vi "5-bit DIO.vi"(0 "DIO Refnum 1":refnum<k21>, 1 "DIO Refnum 2":refnum<k21>, 2 "DIO Refnum 3":refnum<k21>, 3 "DIO Refnum 4":refnum<k21>, 4 "DIO Refnum 5":refnum<k21>, 5 "DIO OUT[4:0]":u8, 7 "DIO DIR[4:0]":u8) -> (17 "DIO IN[4:0]":u8)   [LabVIEW 2019]
panel:
  # "This VI reads a Boolean value from or writes the value to the specified FPGA I/O item according to the direction of the data flow (DIR).\n- DIR: TRUE - Write data to OUT\n- DIR: FALSE - Read data from IN"
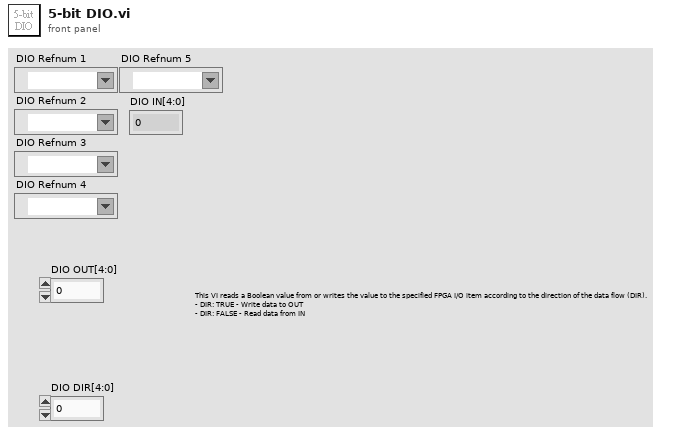
[diagram p1: front panel]
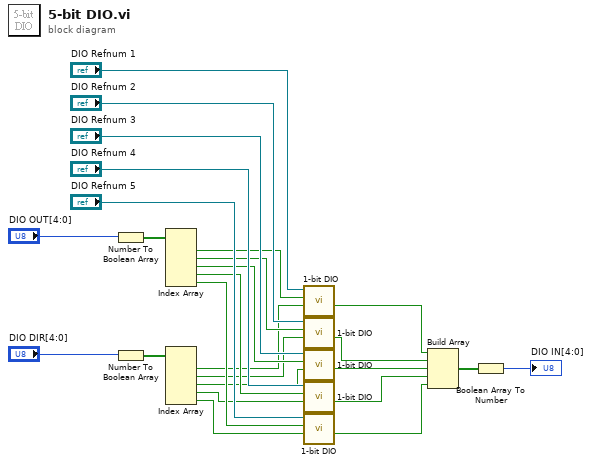
[diagram p0: block diagram]
diagram:
  n1 = Number To Boolean Array(number="DIO OUT[4:0]") -> (Boolean array=w21:bool[])
  n2 = Number To Boolean Array(number="DIO DIR[4:0]") -> (Boolean array=w13:bool[])
  n3 = Index Array(array=w21) -> (element #1=w20:bool, element #2=w19:bool, element #3=w18:bool, element #4=w17:bool, element #5=w16:bool)  [unwired: 5 in]
  n4 = Index Array(array=w13) -> (element #1=w12:bool, element #2=w11:bool, element #3=w10:bool, element #4=w9:bool, element #5=w8:bool)  [unwired: 5 in]
  n5 = call "1-bit DIO.vi"("DIR"=w12, "OUT"=w20, "DIO Refnum"="DIO Refnum 1") -> ("IN"=w7:bool)  [unwired: 8 in]
  n6 = call "1-bit DIO.vi"("DIR"=w11, "OUT"=w19, "DIO Refnum"="DIO Refnum 2") -> ("IN"=w6:bool)  [unwired: 8 in]
  n7 = call "1-bit DIO.vi"("DIR"=w10, "OUT"=w18, "DIO Refnum"="DIO Refnum 3") -> ("IN"=w3:bool)  [unwired: 8 in]
  n8 = call "1-bit DIO.vi"("DIR"=w9, "OUT"=w17, "DIO Refnum"="DIO Refnum 4") -> ("IN"=w4:bool)  [unwired: 8 in]
  n9 = call "1-bit DIO.vi"("DIR"=w8, "OUT"=w16, "DIO Refnum"="DIO Refnum 5") -> ("IN"=w5:bool)  [unwired: 8 in]
  n10 = Build Array(w7, w6, w3, w4, w5) -> (w2:bool[])
  n11 = Boolean Array To Number(Boolean array=w2) -> (number=→"DIO IN[4:0]":u8)
